vi "Example Simple.vi"() -> ()   [LabVIEW 2013]
uses:
  C:/tf/play/labview/Tinkerforge.dll
panel:
  out "touch state":string
  in  "uid":string="fdsg"
  in  "port":i32=4223
  in  "host":string="localhost"
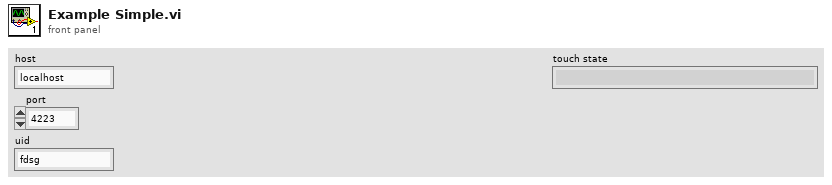
[diagram p1: front panel]
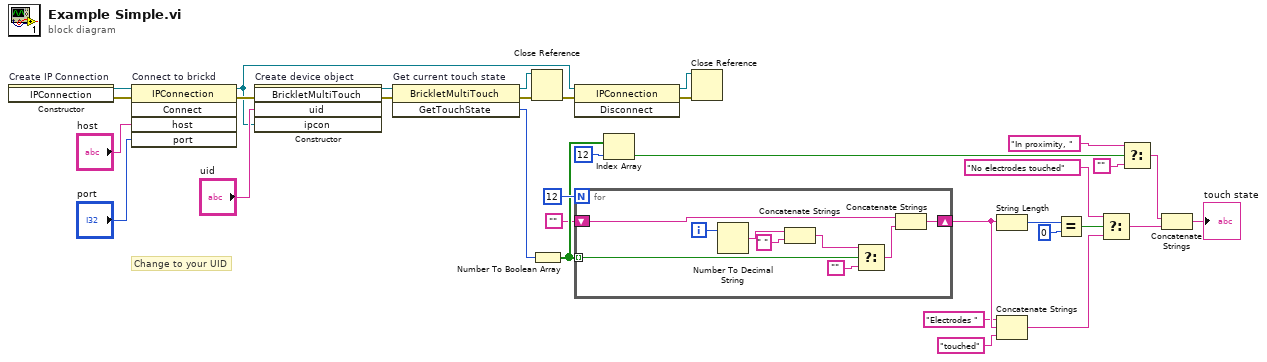
[diagram p0: block diagram]
diagram:
  # "Change to your UID"
  n1 = constructor on="Create IP Connection" class="IPConnection"() -> (reference out=w33:refnum<k24>, error out=w20:errorcluster)  [unwired: 3 in, 1 out]
  n2 = invoke on="Connect to brickd" class="IPConnection" method="Connect"(reference=w33, error in=w20, "host"="host", "port"="port") -> (reference out=w22:refnum<k24>, error out=w29:errorcluster)  [unwired: 1 in, 3 out]
  n3 = constructor on="Create device object" class="BrickletMultiTouch"(error in=w29, "uid"="uid", "ipcon"=w22) -> (reference out=w27:refnum<k24>, error out=w28:errorcluster)  [unwired: 2 in, 3 out]
  n4 = invoke on="Get current touch state" class="BrickletMultiTouch" method="GetTouchState"(reference=w27, error in=w28) -> (reference out=w25:refnum<k24>, error out=w26:errorcluster, "GetTouchState"=w18:i32)  [unwired: 1 in]
  n5 = Close Reference(reference=w25, error in (no error)=w26) -> (error out=w24:errorcluster)
  n6 = Number To Boolean Array(number=w18) -> (Boolean array=w14:bool[])
  n7 = invoke class="IPConnection" method="Disconnect"(reference=w22, error in=w24) -> (reference out=w21:refnum<k24>, error out=w23:errorcluster)  [unwired: 1 in, 1 out]
  n8 = for {
    N: 12 -> [_]
    tunnel: w14 -> [w42] mode=indexing
    shift-right: [w38] -> w7
    shift-left: "" -> [w39]
    i -> [w37]
    n9 = Number To Decimal String(number=w37) -> (decimal integer string=w35:string)  [unwired: 1 in]
    n10 = Concatenate Strings(w35, " " ("string")) -> (w36:string)
    n11 = Select(t=w36, s=w42, f="") -> (s? t:f=w40:string)
    n12 = Concatenate Strings(w39, w40) -> (w38:string)
  }
  n13 = Index Array(array=w14, index=12) -> (element=w15:bool)
  n14 = Close Reference(reference=w21, error in (no error)=w23) -> ()  [unwired: 1 out]
  n15 = String Length(string=w7) -> (length=w11:i32)
  n16 = Concatenate Strings("Electrodes " ("string"), w7, "touched" ("string")) -> (w6:string)
  n17 = Equal?(x=w11, y=0) -> (x = y?=w9:bool)
  n18 = Select(t="No electrodes touched", s=w9, f=w6) -> (s? t:f=w1:string)
  n19 = Select(t="In proximity, ", s=w15, f="") -> (s? t:f=w2:string)
  n20 = Concatenate Strings(w2, w1) -> (→"touch state":string)
